vi "Update Plots Config.vi"(8 "error in (no error)":errorcluster, 10 "Plot Group Config":T1, 11 "Historian Charting Manager in":refnum<class "Historian Charting Manager.lvclass">) -> (0 "error out":errorcluster, 3 "Historian Charting Manager out":refnum<class "Historian Charting Manager.lvclass">)   [LabVIEW 2020, in "VolatusGUI.lvlib" / "Historian Charting Manager.lvclass"]
uses:
  Historian Charting Manager.lvclass
  Historian Charting Manager.lvclass/Historian Charting Manager.ctl
  New Plot Group Data.ctl
  X-Axis Type.ctl
  Scale.ctl
  Plot Config.ctl
  Plot Group Config.ctl
  Plot Group Changed Data.ctl
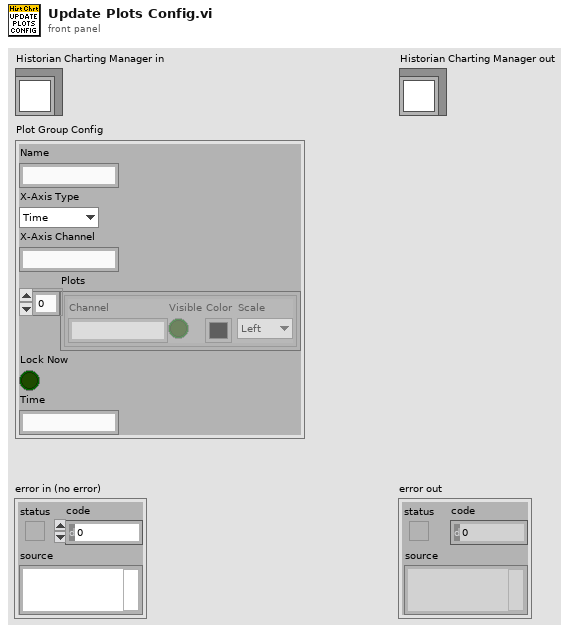
[diagram p1: front panel]
types:
  T1 = typedef "VolatusGUI.lvlib/Historian Charting Manager.lvclass/Plot Group Config.ctl" = cluster{"Name":string, "X-Axis Type":T2, "X-Axis Channel":string, "Plots":T3[], "Lock Now":bool, "Time":string}
  T2 = typedef "VolatusGUI.lvlib/Historian Charting Manager.lvclass/X-Axis Type.ctl" = enum16{"Time", "Channel"}
  T3 = typedef "VolatusGUI.lvlib/Historian Charting Manager.lvclass/Plot Config.ctl" = cluster{"Channel":string, "Visible":bool, "Color":u32, "Scale":T4}
  T4 = typedef "VolatusGUI.lvlib/Historian Charting Manager.lvclass/Scale.ctl" = enum16{"Left", "Right"}
  T5 = typedef "VolatusGUI.lvlib/Historian Charting Manager.lvclass/New Plot Group Data.ctl" = cluster{"Name":string, "Plot Groups":string[]}
  T6 = typedef "VolatusGUI.lvlib/Historian Charting Manager.lvclass/Plot Group Changed Data.ctl" = cluster{"Config":T1}
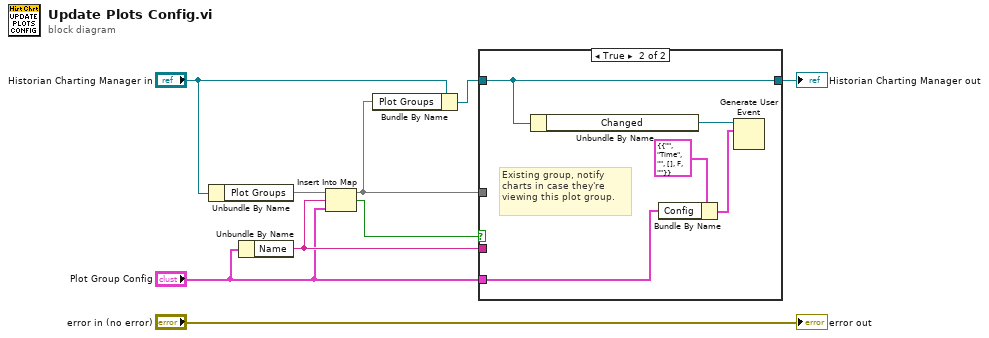
[diagram p0: block diagram]
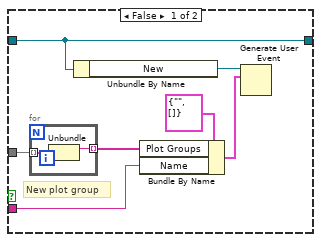
[diagram p2: hidden frame]
diagram:
  n1 = Unbundle By Name("Historian Charting Manager in") -> ("Plot Groups"=w8:map{string, T1})
  n2 = Unbundle By Name("Plot Group Config") -> ("Name"=w7:string)
  n3 = Insert Into Map(map in=w8, key=w7, value="Plot Group Config") -> (map out=w2:map{string, T1}, key already included?=w5:bool)  [unwired: 1 out]
  n4 = Bundle By Name(cluster="Historian Charting Manager in", "Plot Groups"=w2) -> (w3:refnum<class "Historian Charting Manager.lvclass">)
  n5 = case shown="True" w5 {
    tunnel: "Plot Group Config" -> [_ w20]
    tunnel: w7 -> [w11 _]
    tunnel: w3 -> [w10 w19]
    tunnel: w2 -> [w15 _]
    tunnel: [w10 w19] -> w1
    frame False {
      # "New plot group"
      n6 = for {
        tunnel: w15 -> [w18] mode=indexing
        tunnel: [w17] -> w12 mode=indexing
        n7 = Unbundle(w18) -> ("Name"=w17:string)  [unwired: 1 out]
      }
      n8 = Unbundle By Name(w10) -> ("New"=w16:refnum<user-event>)
      n9 = Bundle By Name(cluster=T5 {"Name"="", "Plot Groups"=[]} ("event data"), "Plot Groups"=w12, "Name"=w11) -> (w13:T5)
      n10 = Generate User Event(user event=w16, event data cluster=w13) -> ()  [unwired: 2 in, 2 out]
    }
    frame True {
      # "Existing group, notify charts in case they're viewing this plot group."
      n11 = Unbundle By Name(w19) -> ("Changed"=w23:refnum<user-event>)
      n12 = Bundle By Name(cluster=T6 {"Config"={"Name"="", "X-Axis Type"=enum."Time", "X-Axis Channel"="", "Plots"=[], "Lock Now"=FALSE, "Time"=""}} ("event data"), "Config"=w20) -> (w21:T6)
      n13 = Generate User Event(user event=w23, event data cluster=w21) -> ()  [unwired: 2 in, 2 out]
    }
  }
  "Historian Charting Manager out" <- w1
  "error out" <- "error in (no error)"
